vi "Charger_Single Channel.vi"(6 "Stop Refnum":refnum<vi>, 7 "Status Refnum":T1, 8 "error in":errorcluster, 9 "semaphore":T2) -> (0 "error out":errorcluster)   [LabVIEW 2020]
uses:
  Charger_Status Refnum.ctl
  Drivers/Charger Test Set/Charger_Input Control.ctl
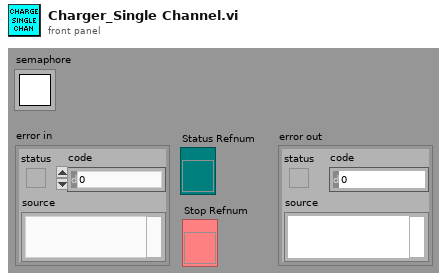
[diagram p1: front panel]
types:
  T1 = typedef "Charger_Status Refnum.ctl" = refnum<vi>
  T2 = typedef "Semaphore RefNum" = refnum<k1>
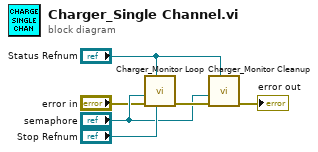
[diagram p0: block diagram]
diagram:
  n1 = call "Charger_Monitor Loop.vi"("Stop Refnum"="Stop Refnum", "Status Refnum"="Status Refnum", "error in"="error in", "semaphore"="semaphore") -> ("error out"=w4:errorcluster)  [unwired: 6 in, 1 out]
  n2 = call "Charger_Monitor Cleanup.vi"("Status Refnum"="Status Refnum", "error in"=w4, "semaphore"="semaphore") -> ("error out"=→"error out":errorcluster)  [unwired: 5 in, 1 out]
